vi "Dispatch PVMonitors.vi"(4 "PV Activate Queue":refnum<queue>, 6 "PV Data Queue":refnum<queue>, 8 "Error In":errorcluster, 11 "CS++PVProxy in":refnum<class "CS++PVProxy.lvclass">) -> (0 "Error Out":errorcluster, 3 "CS++PVProxy out":refnum<class "CS++PVProxy.lvclass">)   [LabVIEW 2016, in "CS++PVProxy.lvlib" / "CS++PVProxy.lvclass"]
doc: "Dispatch nested PVMonitor actors according to PV protocoll prefix."
uses:
  CS++PVProxy.lvclass
  C:/User/Brand/LVP/CSPP/Packages/CSPP_Core/Actors/CS++BaseActor/CS++BaseActor.lvclass
  C:/Program Files (x86)/National Instruments/LabVIEW 2016/vi.lib/ActorFramework/Actor/Actor.lvclass
  CS++PVMonitor/CS++PVMonitor.lvclass
  CS++GUIActor Messages/Update-PV Msg/Update-PV Msg.lvclass
  C:/User/Brand/LVP/CSPP/Packages/CSPP_Core/Actors/CS++PVMonitor Messages/CS++PVUpdate Msg/CS++PVUpdate Msg.lvclass
  CS++BaseActor/CS++BaseActor.lvclass/CS++BaseActor.ctl
  CS++PVProxy.lvclass/CS++PVProxy.ctl
  CS++PVMonitor Messages/CS++PVUpdate Msg/CS++PVUpdate Msg.lvclass/CS++PVUpdate Msg.ctl
  Classes/CS++ProcessVariables/ProcessVariable/PV.lvclass/PV.ctl
  CS++PVMonitor/CS++PVMonitor.lvclass/CS++PVMonitor.ctl
  <vilib>/ActorFramework/Actor/Actor.lvclass/Actor.ctl
  <vilib>/ActorFramework/Message Enqueuer/Message Enqueuer.lvclass/Message Enqueuer.ctl
  CS++PVMonitor Messages/Register PVs Msg/Register PVs Msg.lvclass/Register PVs Msg.ctl
  Read DelayedActivation.vi
  <vilib>/ActorFramework/Message Enqueuer/Init from Existing Queue.vi
  <vilib>/ActorFramework/Message Enqueuer/Enqueue.vi
  CS++PVMonitor Messages/Register PVs Msg/Register PVs Msg.lvclass
  C:/Program Files (x86)/National Instruments/LabVIEW 2016/vi.lib/ActorFramework/Message/Message.lvclass
  <vilib>/ActorFramework/Message Priority Queue/Priority Enqueue.vi
  CS++PVMonitor Messages/CS++PVUpdate Msg/CS++PVUpdate Msg.lvclass
  Classes/CS++ProcessVariables/PVConnection/PVConnection.lvclass
  Classes/CS++ProcessVariables/ProcessVariable/PV.lvclass
  <vilib>/ActorFramework/Message Enqueuer/Message Enqueuer.lvclass
  CS++BaseActor/CS++BaseActor.lvclass
  <vilib>/ActorFramework/Actor/Actor.lvclass
  Libraries/Base/CS++Base.lvlib
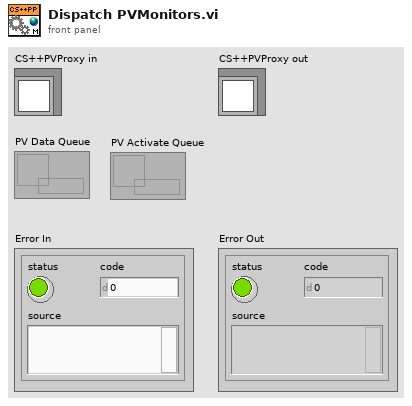
[diagram p1: front panel]
types:
  T1 = cluster{"Msgs":refnum<class "Update-PV Msg.lvclass">[]}[]
  T2 = cluster{"Name":string, "Polling-String":string, "CS++PVUpdate Msg":refnum<class "CS++PVUpdate Msg.lvclass">, "PVConnection":refnum<class "PVConnection.lvclass">}[]
  T3 = cluster{"Msgs":refnum<class "CS++PVUpdate Msg.lvclass">[]}
  T4 = cluster{"Msgs":refnum<class "CS++PVUpdate Msg.lvclass">[]}[]
  T5 = cluster{refnum<class "CS++PVUpdate Msg.lvclass">[]}
  T6 = cluster{"Worker Actor's Enqueuer":refnum<class "Message Enqueuer.lvclass">, "Msgs":refnum<class "CS++PVUpdate Msg.lvclass">[]}
  T7 = cluster{"Self Enqueuer":refnum<class "Message Enqueuer.lvclass">, "Msgs":refnum<class "CS++PVUpdate Msg.lvclass">[]}
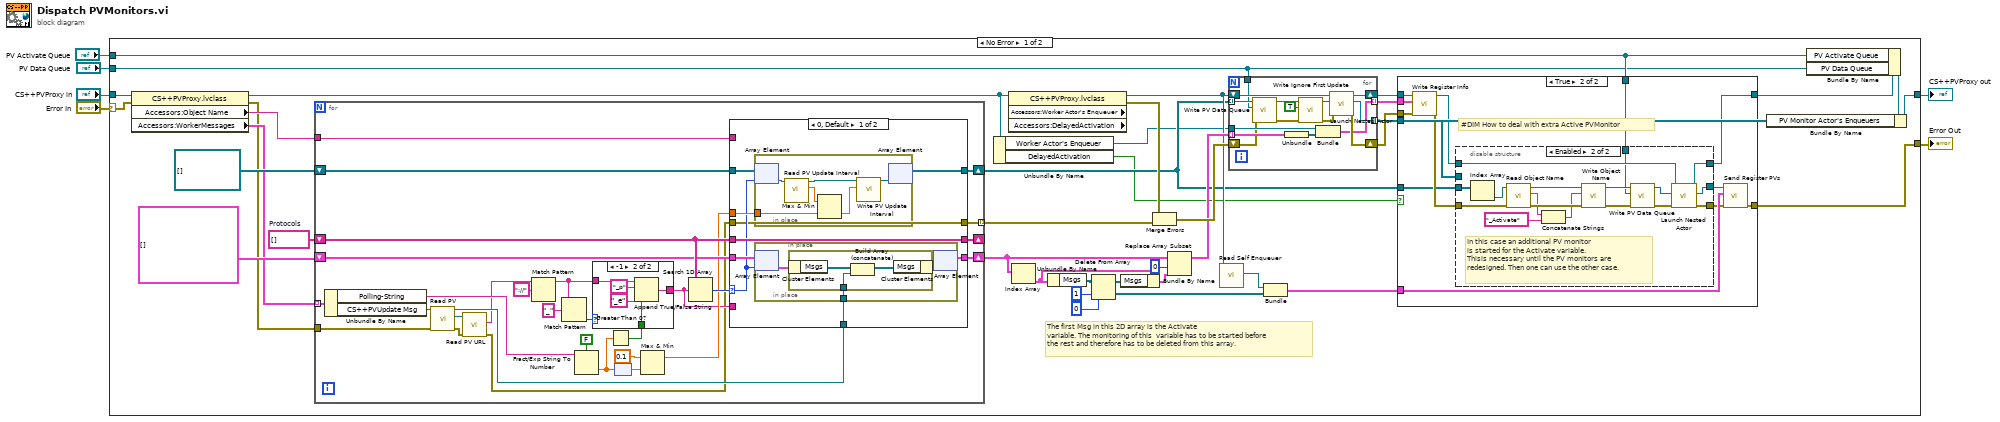
[diagram p0: block diagram]
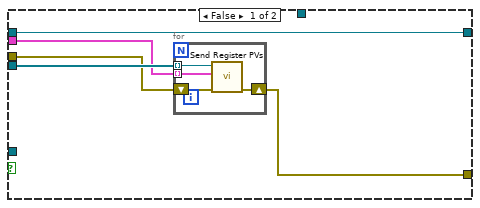
[diagram p2: hidden frame]
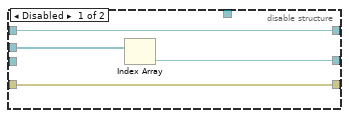
[diagram p3: hidden frame]
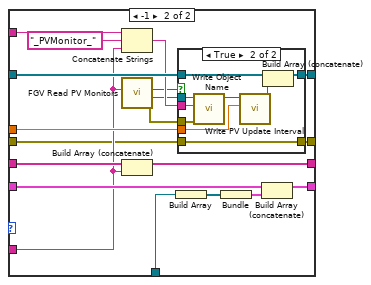
[diagram p5: hidden frame]
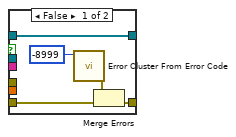
[diagram p6: hidden frame]
diagram:
  n1 = case shown="No Error" "Error In" {
    selector: "Error In" -> [w42 w194]
    tunnel: [w30 w194] -> w5
    tunnel: [w43 w193] -> w3
    tunnel: "CS++PVProxy in" -> [w44 w193]
    tunnel: "PV Data Queue" -> [w10 _]
    tunnel: "PV Activate Queue" -> [w11 _]
    frame No Error {
      w40 = string[] []  # Protocols
      # "The first Msg in this 2D array is the Activate\nvariable. The monitoring of this  variable has to be started before\nthe rest and therefore has to be deleted from this array."
      n2 = property class="CS++PVProxy.lvclass"(reference=w44, error in=w42) -> (reference out=w9:refnum<class "CS++PVProxy.lvclass">, error out=w33:errorcluster, "Accessors:Object Name"=w36:string, "Accessors:WorkerMessages"=w34:T2)
      n3 = for {
        shift-right: [w132] -> w23
        shift-left: refnum<class "CS++PVMonitor.lvclass">[] [] -> [w129]
        shift-right: [w131] -> _
        shift-left: w40 -> [w130]
        tunnel: w36 -> [w128]
        shift-right: [w126] -> w27
        shift-left: T1 [] -> [w127]
        tunnel: [w125] -> w37 mode=indexing
        tunnel: w34 -> [w115] mode=indexing
        tunnel: w33 -> [w107]
        n4 = Unbundle By Name(w115) -> ("Polling-String"=w114:string, "CS++PVUpdate Msg"=w113:refnum<class "CS++PVUpdate Msg.lvclass">)
        n5 = call "Read PV.vi"("error in (no error)"=w107, "CS++PVUpdate Msg in"=w113) -> ("error out"=w109:errorcluster, "PV"=w111:refnum<class "PV.lvclass">, "CS++PVUpdate Msg out"=w112:refnum<class "CS++PVUpdate Msg.lvclass">)  [unwired: 7 in]
        n6 = call "Read PV URL.vi"("error in (no error)"=w109, "PV in"=w111) -> ("error out"=w108:errorcluster, "PV URL"=w110:string)  [unwired: 7 in, 1 out]
        n7 = Match Pattern(string=w110, regular expression="://") -> (before substring=w106:string)  [unwired: 1 in, 3 out]
        n8 = Match Pattern(string=w106, regular expression="_") -> (offset past match=w104:i32)  [unwired: 1 in, 3 out]
        n9 = Fract/Exp String To Number(use system decimal point (T)=FALSE, string=w114) -> (number=w119:dbl)  [unwired: 2 in, 1 out]
        n10 = Greater Than 0?(x=w119) -> (x > 0?=w116:bool)
        n11 = case shown="-1" w104 {
          tunnel: [w133 w138] -> w117
          tunnel: w116 -> [_ w137]
          tunnel: w106 -> [w133 w134]
          frame 0, Default {
          }
          frame -1 {
            n12 = Append True/False String(1:w137, 2:"_e" ("false string"), 3:"_p" ("true string"), 4:w134) -> (0:w138:string)
          }
        }
        n13 = node(w119) -> (w121:dbl[unit])
        n14 = Max & Min(x=dbl[unit] 0.1, y=w121) -> (max(x,y)=w118:dbl[unit])  [unwired: 1 out]
        n15 = Search 1D Array(1D array=w130, element=w117) -> (index of element=w122:i32)  [unwired: 1 in]
        n16 = case shown="0, Default" w122 {
          selector: w122 -> [w142 _]
          tunnel: [w145 w178] -> w132
          tunnel: [w147 w177] -> w131
          tunnel: w117 -> [_ w165]
          tunnel: w130 -> [w147 w176]
          tunnel: w129 -> [w146 w175]
          tunnel: w118 -> [w144 w172]
          tunnel: w128 -> [_ w171]
          tunnel: w112 -> [w141 w170]
          tunnel: w127 -> [w143 w168]
          tunnel: [w140 w166] -> w126
          tunnel: w108 -> [w139 w162]
          tunnel: [w139 w160] -> w125
          frame 0, Default {
            n17 = in-place {
              in-place-border: w144 -> [w159]
              n18 = in-place-array #1(w146, w142) -> (w156:refnum<class "CS++PVMonitor.lvclass">)
              n19 = call "Read PV Update Interval.vi"("CS++PVMonitor in"=w156) -> ("PV Update Interval"=w154:dbl[unit], "CS++PVMonitor out"=w155:refnum<class "CS++PVMonitor.lvclass">)  [unwired: 8 in, 1 out]
              n20 = Max & Min(x=w154, y=w159) -> (min(x,y)=w158:dbl[unit])  [unwired: 1 out]
              n21 = call "Write PV Update Interval.vi"("PV Update Interval"=w158, "CS++PVMonitor in"=w155) -> ("CS++PVMonitor out"=w157:refnum<class "CS++PVMonitor.lvclass">)  [unwired: 8 in, 1 out]
              n22 = in-place-array #1(w157) -> (w145:refnum<class "CS++PVMonitor.lvclass">[])  [unwired: 1 out]
            }
            n23 = in-place {
              in-place-border: w141 -> [w148]
              n24 = in-place-array #2(w143, w142) -> (w150:T3)
              n25 = in-place {
                in-place-border: w148 -> [w152]
                n26 = in-place-cluster #3(w150) -> ("Msgs"=w153:refnum<class "CS++PVUpdate Msg.lvclass">[])
                n27 = Build Array (concatenate)(w153, w152) -> (w151:refnum<class "CS++PVUpdate Msg.lvclass">[])
                n28 = in-place-cluster #3("Msgs"=w151) -> (w149:T3)
              }
              n29 = in-place-array #2(w149) -> (w140:T4)  [unwired: 1 out]
            }
          }
          frame -1 {
            n30 = Concatenate Strings(w171, "_PVMonitor_" ("Object Name"), w165) -> (w173:string)
            n31 = call "FGV Read PV Monitors.vi"("PV Monitor"=w165) -> ("Error Out"=w163:errorcluster, "CS++PVMonitor"=w164:refnum<class "CS++PVMonitor.lvclass">, "Success"=w161:bool)  [unwired: 6 in, 2 out]
            n32 = Build Array (concatenate)(w176, w165) -> (w177:string[])
            n33 = Build Array(w170) -> (w169:refnum<class "CS++PVUpdate Msg.lvclass">[])
            n34 = case shown="True" w161 {
              tunnel: [w183 w192] -> w178
              tunnel: w175 -> [w183 w191]
              tunnel: w173 -> [_ w190]
              tunnel: w172 -> [_ w185]
              tunnel: w164 -> [_ w189]
              tunnel: w163 -> [_ w188]
              tunnel: w162 -> [w182 w187]
              tunnel: [w181 w187] -> w160
              frame False {
                n35 = call <vilib>:"Error Cluster From Error Code.vi"("error code (0)"=-8999) -> ("error out"=w180:errorcluster)  [unwired: 8 in]
                n36 = Merge Errors(w180, w182) -> (w181:errorcluster)
              }
              frame True {
                n37 = call "Write Object Name.vi"("error in (no error)"=w188, "Object Name"=w190, "CS++BaseActor in"=w189) -> ("CS++BaseActor out"=w186:refnum<class "CS++PVMonitor.lvclass">)  [unwired: 7 in, 1 out]
                n38 = call "Write PV Update Interval.vi"("PV Update Interval"=w185, "CS++PVMonitor in"=w186) -> ("CS++PVMonitor out"=w184:refnum<class "CS++PVMonitor.lvclass">)  [unwired: 8 in, 1 out]
                n39 = Build Array (concatenate)(w191, w184) -> (w192:refnum<class "CS++PVMonitor.lvclass">[])
              }
            }
            n40 = Bundle(w169) -> (w167:T5)  [unwired: 1 in]
            n41 = Build Array (concatenate)(w168, w167) -> (w166:T4)
          }
        }
      }
      n42 = Unbundle By Name(w9) -> ("Worker Actor's Enqueuer"=w8:refnum<class "Message Enqueuer.lvclass">, "DelayedActivation"=w7:bool)
      n43 = property class="CS++PVProxy.lvclass" props=["Accessors:Worker Actor's Enqueuer", "Accessors:DelayedActivation"](reference=w9) -> (reference out=w25:refnum<class "CS++PVProxy.lvclass">, error out=w35:errorcluster)  [unwired: 1 in, 2 out]
      n44 = Index Array(array=w27) -> (element=w20:T3)  [unwired: 1 in]
      n45 = Unbundle By Name(w20) -> ("Msgs"=w22:refnum<class "CS++PVUpdate Msg.lvclass">[])
      n46 = Delete From Array(array=w22, length=1, index=0) -> (deleted portion=w15:refnum<class "CS++PVUpdate Msg.lvclass">[], array with subset deleted=w19:refnum<class "CS++PVUpdate Msg.lvclass">[])
      n47 = Bundle By Name(cluster=w20, "Msgs"=w19) -> (w18:T3)
      n48 = Merge Errors(w35, w37) -> (w39:errorcluster)
      n49 = Replace Array Subset(array=w27, new element=w18, index=0) -> (w26:T4)
      n50 = call <vilib>:"Read Self Enqueuer.vi"("Actor"=w25) -> ("Self Enqueuer"=w16:refnum<class "Message Enqueuer.lvclass">)  [unwired: 10 in]
      n51 = for {
        tunnel: w8 -> [w103]
        tunnel: w23 -> [w95] mode=indexing
        tunnel: w26 -> [w102] mode=indexing
        tunnel: [w99] -> w29 mode=indexing
        shift-right: [w97] -> w31
        shift-left: w39 -> [w94]
        shift-right: [w98] -> w32
        shift-left: w25 -> [w101]
        tunnel: [w96] -> w28 mode=indexing
        tunnel: w10 -> [w93]
        n52 = call-dynamic "Write PV Data Queue.vi"("error in (no error)"=w94, "Data Queue"=w93, "CS++PVMonitor in"=w95) -> ("error out"=w90:errorcluster, "CS++PVMonitor out"=w92:refnum<class "CS++PVMonitor.lvclass">)  [unwired: 7 in]
        n53 = Unbundle(w102) -> ("Msgs"=w100:refnum<class "CS++PVUpdate Msg.lvclass">[])
        n54 = call "Write Ignore First Update.vi"("error in (no error)"=w90, "Ignore First Update"=TRUE, "CS++PVMonitor in"=w92) -> ("error out"=w89:errorcluster, "CS++PVMonitor out"=w91:refnum<class "CS++PVMonitor.lvclass">)  [unwired: 7 in]
        n55 = Bundle("Worker Actor's Enqueuer"=w103, "Msgs"=w100) -> (w96:T6)  [unwired: 1 in]
        n56 = call <vilib>:"Launch Nested Actor.vi"("error in (no error)"=w89, "Nested Actor"=w91, "Caller Actor in"=w101) -> ("error out"=w97:errorcluster, "Nested Actor's Enqueuer"=w99:refnum<class "Message Enqueuer.lvclass">, "Caller Actor out"=w98:refnum<class "CS++PVProxy.lvclass">)  [unwired: 6 in]
      }
      n57 = Bundle("Self Enqueuer"=w16, "Msgs"=w15) -> (w24:T7)  [unwired: 1 in]
      n58 = case shown="True" w7 {
        tunnel: w32 -> [w45 w66]
        tunnel: w31 -> [w47 w65]
        tunnel: [w46 w64] -> w30
        tunnel: w29 -> [w49 w55]
        tunnel: w28 -> [w48 w62]
        tunnel: w24 -> [_ w61]
        tunnel: [w45 w57] -> w12
        tunnel: w23 -> [_ w56]
        tunnel: w11 -> [_ w54]
        frame False {
          n59 = for {
            tunnel: w49 -> [w53] mode=indexing
            tunnel: w48 -> [w52] mode=indexing
            shift-right: [w50] -> w46
            shift-left: w47 -> [w51]
            n60 = call "Send Register PVs.vi"("error in (no error)"=w51, "Register Info"=w52, "Message Enqueuer"=w53) -> ("error out"=w50:errorcluster)  [unwired: 7 in, 1 out]
          }
        }
        frame True {
          # "#DIM How to deal with extra Active PVMonitor"
          n61 = call "Write Register Info.vi"("error in (no error)"=w65, "Register Info"=w62, "CS++PVProxy in"=w66) -> ("error out"=w60:errorcluster, "CS++PVProxy out"=w58:refnum<class "CS++PVProxy.lvclass">)  [unwired: 7 in]
          n62 = disable-structure shown="Enabled" {
            disable-tunnel: w55 -> [w70 _]
            disable-tunnel: [w69 w87] -> w63
            disable-tunnel: w60 -> [w68 w79]
            disable-tunnel: [w68 w86] -> w59
            disable-tunnel: w58 -> [w67 w85]
            disable-tunnel: [w67 w84] -> w57
            disable-tunnel: w56 -> [_ w83]
            disable-tunnel: w54 -> [_ w71]
            frame Disabled {
              n63 = Index Array(array=w70) -> (element=w69:refnum<class "Message Enqueuer.lvclass">)  [unwired: 1 in]
            }
            frame Enabled {
              # "In this case an additional PV monitor\nis started for the Activate variable.\nThisis necessary until the PV monitors are\nredesigned. Then one can use the other case."
              n64 = Index Array(array=w83) -> (element=w80:refnum<class "CS++PVMonitor.lvclass">)  [unwired: 1 in]
              n65 = call "Read Object Name.vi"("error in (no error)"=w79, "CS++BaseActor in"=w80) -> ("error out"=w82:errorcluster, "Object Name"=w77:string, "CS++BaseActor out"=w81:refnum<class "CS++PVMonitor.lvclass">)  [unwired: 7 in]
              n66 = Concatenate Strings(w77, "_Activate" ("string")) -> (w78:string)
              n67 = call "Write Object Name.vi"("error in (no error)"=w82, "Object Name"=w78, "CS++BaseActor in"=w81) -> ("error out"=w73:errorcluster, "CS++BaseActor out"=w75:refnum<class "CS++PVMonitor.lvclass">)  [unwired: 7 in]
              n68 = call-dynamic "Write PV Data Queue.vi"("error in (no error)"=w73, "Data Queue"=w71, "CS++PVMonitor in"=w75) -> ("error out"=w72:errorcluster, "CS++PVMonitor out"=w74:refnum<class "CS++PVMonitor.lvclass">)  [unwired: 7 in]
              n69 = call <vilib>:"Launch Nested Actor.vi"("error in (no error)"=w72, "Nested Actor"=w74, "Caller Actor in"=w85) -> ("error out"=w86:errorcluster, "Nested Actor's Enqueuer"=w87:refnum<class "Message Enqueuer.lvclass">, "Caller Actor out"=w84:refnum<class "CS++PVProxy.lvclass">)  [unwired: 6 in]
            }
          }
          n70 = call "Send Register PVs.vi"("error in (no error)"=w59, "Register Info"=w61, "Message Enqueuer"=w63) -> ("error out"=w64:errorcluster)  [unwired: 7 in, 1 out]
        }
      }
      n71 = Bundle By Name(cluster=w12, "PV Activate Queue"=w11, "PV Data Queue"=w10) -> (w13:refnum<class "CS++PVProxy.lvclass">)
      n72 = Bundle By Name(cluster=w13, "PV Monitor Actor's Enqueuers"=w29) -> (w43:refnum<class "CS++PVProxy.lvclass">)
    }
    frame Error {
    }
  }
  "Error Out" <- w5
  "CS++PVProxy out" <- w3
